vi "Data_Read_Signal_From_Disk_Start_End.vi"(4 "End":i32, 6 "Start":i32, 8 "error in (no error)":errorcluster, 9 "filename":string, 10 "path":path, 11 "wfm info":T1) -> (0 "error out":errorcluster, 2 "data":i16[](array[numeric]), 5 "wfm info":T1)   [LabVIEW 2017]
doc: "This VI reads a raw dataset from a disk file with the following format :\n- number of points = one value (I32)\n- data = number of points * values (I16)\n- 1/sample rate, i.e. time step = one value (SGL or F32)\n- vertical range = one value (SGL)\n- offset = one value (SGL)\nCalibrated data are obtained with : data * vertical range + offset"
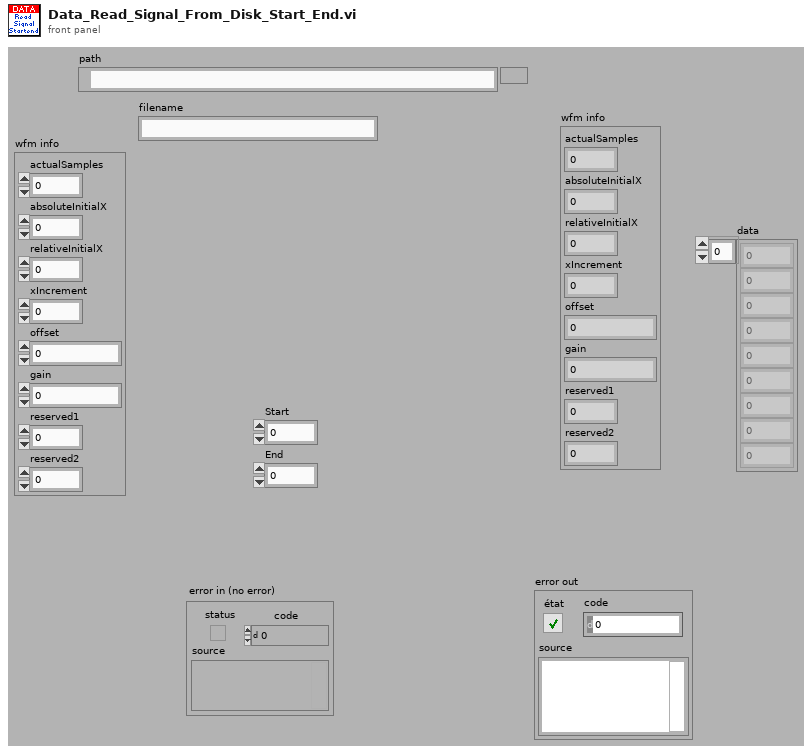
[diagram p1: front panel]
types:
  T1 = cluster{"actualSamples":i32, "absoluteInitialX":dbl, "relativeInitialX":dbl, "xIncrement":dbl, "offset":dbl, "gain":dbl, "reserved1":dbl, "reserved2":dbl}
  T2 = enum16{"big-endian, network order", "native, host order", "little-endian"}
  T3 = enum16{"open", "replace", "create", "open or create", "replace or create", "replace or create with confirmation"}
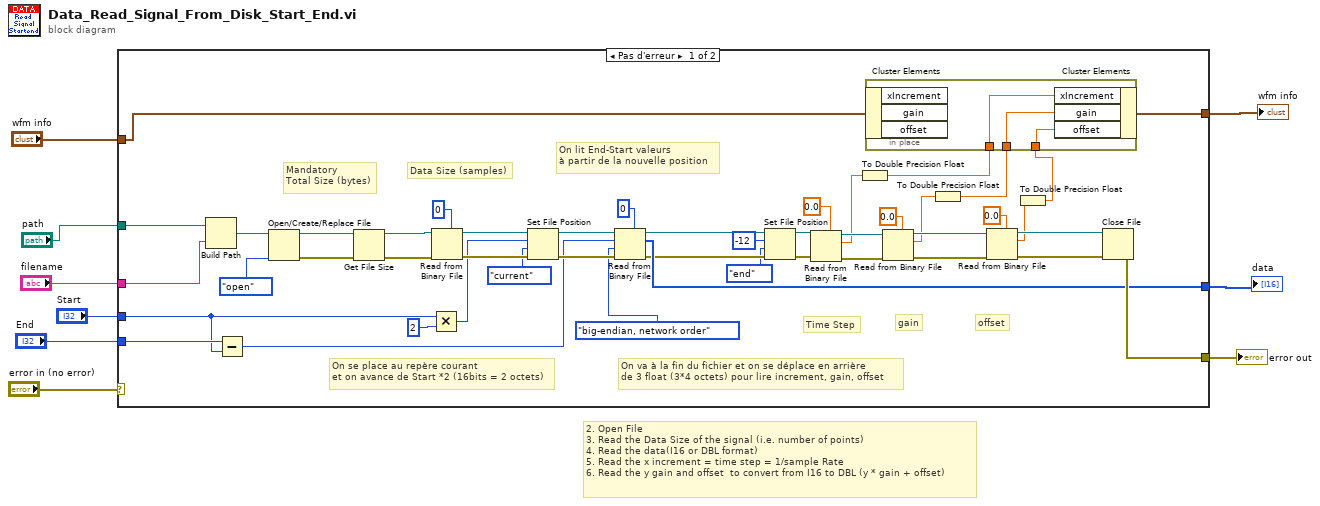
[diagram p0: block diagram]
diagram:
  # "2. Open File\n3. Read the Data Size of the signal (i.e. number of points)\n4. Read the data(I16 or DBL format)\n5. Read the x increment = time step = 1/sample Rate\n6. Read the y gain and offset  to convert from I16 to DBL (y * gain + offset)"
  n1 = case shown="Pas d'erreur" "error in (no error)" {
    selector: "error in (no error)" -> [_ w60]
    tunnel: [w55 w60] -> w7
    tunnel: "wfm info" -> [w37 w59]
    tunnel: "path" -> [w52 _]
    tunnel: "filename" -> [w51 _]
    tunnel: [w44 _] -> w3
    tunnel: [w35 w59] -> w4
    tunnel: "Start" -> [w11 _]
    tunnel: "End" -> [w12 _]
    frame No Error {
      # "On va à la fin du fichier et on se déplace en arrière\nde 3 float (3*4 octets) pour lire increment, gain, offset"
      # "On lit End-Start valeurs\nà partir de la nouvelle position"
      # "On se place au repère courant\net on avance de Start *2 (16bits = 2 octets)"
      # "gain"
      # "Time Step"
      # "offset"
      # "Data Size (samples)"
      # "Mandatory\nTotal Size (bytes)"
      n2 = Build Path(base path=w52, name or relative path=w51) -> (appended path=w53:path)
      n3 = Subtract(x=w12, y=w11) -> (x-y=w10:i32)
      n4 = Open/Create/Replace File(file path (use dialog)=w53, operation (0:open)=T3."open" ("opération (0 : open)")) -> (refnum out=w46:refnum<file>, error out=w45:errorcluster)  [unwired: 4 in, 1 out]
      n5 = Get File Size(file=w46, error in=w45) -> (refnum out=w49:refnum<file>, 0:w48:errorcluster)  [unwired: 1 out]
      n6 = Multiply(x=w11, y=2) -> (x*y=w13:i32)
      n7 = Read from Binary File(5:0, 8:w48, 11:w49) -> (0:w30:errorcluster, 3:w47:refnum<file>)  [unwired: 3 in, 2 out]
      n8 = Set File Position(offset (in bytes) (0)=w13, refnum=w47, from (0:start)=enum16{"start", "end", "current"}."current" ("à partir de (0 : start)"), error in=w30) -> (refnum out=w31:refnum<file>, error out=w29:errorcluster)
      n9 = Read from Binary File(5:i16 0, 8:w29, 9:T2."big-endian, network order" ("ordre des octets (0 : big-Endian, network order)"), 10:w10, 11:w31) -> (0:w18:errorcluster, 2:w44:i16[], 3:w40:refnum<file>)  [unwired: 1 in, 1 out]
      n10 = Set File Position(offset (in bytes) (0)=i64 -12 ("offset (en octets) (0)"), refnum=w40, from (0:start)=enum16{"start", "end", "current"}."end" ("à partir de (0 : start)"), error in=w18) -> (refnum out=w19:refnum<file>, error out=w17:errorcluster)
      n11 = Read from Binary File(5:sgl 0.0 ("type de données"), 8:w17, 11:w19) -> (0:w26:errorcluster, 2:w22:sgl, 3:w23:refnum<file>)  [unwired: 3 in, 1 out]
      n12 = To Double Precision Float(number=w22) -> (double precision float=w34:dbl)
      n13 = Read from Binary File(5:sgl 0.0 ("type de données"), 8:w26, 11:w23) -> (0:w42:errorcluster, 2:w24:sgl, 3:w43:refnum<file>)  [unwired: 3 in, 1 out]
      n14 = To Double Precision Float(number=w24) -> (double precision float=w33:dbl)
      n15 = Read from Binary File(5:sgl 0.0, 8:w42, 11:w43) -> (0:w38:errorcluster, 2:w36:sgl, 3:w39:refnum<file>)  [unwired: 3 in, 1 out]
      n16 = To Double Precision Float(number=w36) -> (double precision float=w32:dbl)
      n17 = in-place {
        in-place-border: w32 -> [w58]
        in-place-border: w33 -> [w57]
        in-place-border: w34 -> [w56]
        n18 = in-place-cluster #1(w37) -> ()  [unwired: 3 out]
        n19 = in-place-cluster #1("xIncrement"=w56, "gain"=w57, "offset"=w58) -> (w35:T1)
      }
      n20 = Close File(refnum=w39, error in=w38) -> (error out=w55:errorcluster)  [unwired: 1 out]
    }
    frame Error {
    }
  }
  "error out" <- w7
  "data" <- w3
  "wfm info" <- w4
